vi "CALC_DATA_CUST.vi"(0 "VISA IN":refnum<visa-resource-name>, 1 "Buffer Name":string, 2 "Data":string, 5 "error in":errorcluster, 7 "Channel":i32) -> (14 "VISA Out":refnum<visa-resource-name>, 19 "error out":errorcluster)   [LabVIEW 2018, in "PNA-X.lvlib"]
doc: "CALCulate<cnum>:DATA:CUSTom <name>,<data> \n(Read-Write) Reads or writes data from a custom-named measurement buffer. \nSee Critical Note \nParameters \n<cnum> Channel number of the measurement. There must be a selected measurement \non that channel. If unspecified, <cnum> is set to 1. \n<name> Name of the buffer to be read or written \n<data> Data to be read or written to the custom buffer. Format as one number per data \npoint. \nExamples CALC:DATA:CUST 'VectorResult0',0,1,2,3,4,5 'Write \nCALC:DATA:CUST? 'VectorResult0' 'Read \nQuery Syntax CALCulate:DATA:CUSTom? <name> \nReturn Type Depends on Form:Data \nDefault Not Applicable"
uses:
  PNA-X.lvlib
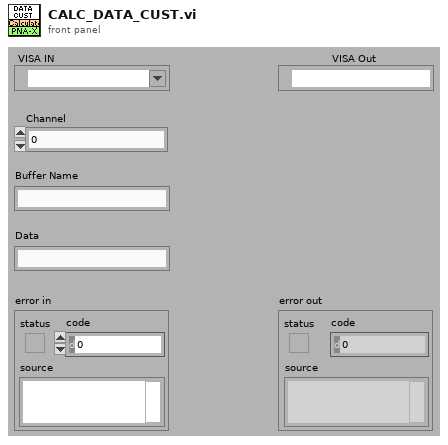
[diagram p1: front panel]
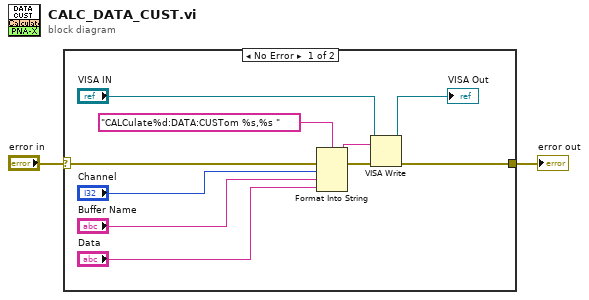
[diagram p0: block diagram]
diagram:
  n1 = case shown="No Error" "error in" {
    selector: "error in" -> [w12 w13]
    tunnel: [w7 w13] -> w1
    frame No Error {
      n2 = Format Into String(format string="CALCulate%d:DATA:CUSTom %s,%s " ("Cmdline"), error in=w12, "Channel", "Buffer Name", "Data") -> (resulting string=w10:string, error out=w11:errorcluster)  [unwired: 1 in]
      n3 = VISA Write(VISA resource name="VISA IN", write buffer=w10, error in (no error)=w11) -> (VISA resource name out=→"VISA Out":refnum<visa-resource-name>, error out=w7:errorcluster)  [unwired: 1 out]
    }
    frame Error {
    }
  }
  "error out" <- w1
